vi "GeoData.vi"() -> ()   [LabVIEW 2017] (continued)
\n76008\t48367\tAledo\tTX\tParker County\tH1\n79035\t48369\tFriona\tTX\tParmer County\tH1\n79325\t48369\tFarwell\tTX\tParmer County\tH1\n79009\t48369\tBovina\tTX\tParmer County\tH1\n79347\t48369\tMuleshoe\tTX\tParmer County\tH1\n79053\t48369\tLazbuddie\tTX\tParmer County\tH1\n79740\t48371\tGirvin\tTX\tPecos County\tH1\n79735\t48371\tFort stockton\tTX\tPecos County\tH1\n79743\t48371\tImperial\tTX\tPecos County\tH1\n79781\t48371\tSheffield\tTX\tPecos County\tH1\n79730\t48371\tCoyanosa\tTX\tPecos County\tH1\n79744\t48371\tIraan\tTX\tPecos County\tH1\n77350\t48373\tLeggett\tTX\tPolk County\tH1\n77326\t48373\tAce\tTX\tPolk County\tH1\n75936\t48373\tChester\tTX\tPolk County\tH1\n77332\t48373\tDallardsville\tTX\tPolk County\tH1\n77327\t48373\tCleveland\tTX\tPolk County\tH1\n75960\t48373\tMoscow\tTX\tPolk County\tH1\n77360\t48373\tOnalaska\tTX\tPolk County\tH1\n77351\t48373\tLivingston\tTX\tPolk County\tH1\n75934\t48373\tCamden\tTX\tPolk County\tH1\n75939\t48373\tCorrigan\tTX\tPolk County\tH1\n77335\t48373\tGoodrich\tTX\tPolk County\tH1\n77399\t48373\tLivingston\tTX\tPolk County\tH1\n79103\t48375\tAmarillo\tTX\tPotter County\tH1\n79116\t48375\tAmarillo\tTX\tPotter County\tH1\n79012\t48375\tBushland\tTX\tPotter County\tH1\n79106\t48375\tAmarillo\tTX\tPotter County\tH1\n79102\t48375\tAmarillo\tTX\tPotter County\tH1\n79068\t48375\tPanhandle\tTX\tPotter County\tH1\n79108\t48375\tAmarillo\tTX\tPotter County\tH1\n79105\t48375\tAmarillo\tTX\tPotter County\tH1\n79107\t48375\tAmarillo\tTX\tPotter County\tH1\n79124\t48375\tAmarillo\tTX\tPotter County\tH1\n79159\t48375\tAmarillo\tTX\tPotter County\tH1\n79098\t48375\tWildorado\tTX\tPotter County\tH1\n79058\t48375\tMasterson\tTX\tPotter County\tH1\n79120\t48375\tAmarillo\tTX\tPotter County\tH1\n79117\t48375\tAmarillo\tTX\tPotter County\tH1\n79118\t48375\tAmarillo\tTX\tPotter County\tH1\n79111\t48375\tAmarillo\tTX\tPotter County\tH1\n79101\t48375\tAmarillo\tTX\tPotter County\tH1\n79109\t48375\tAmarillo\tTX\tPotter County\tH1\n79121\t48375\tAmarillo\tTX\tPotter County\tH1\n79104\t48375\tAmarillo\tTX\tPotter County\tH1\n79845\t48377\tPresidio\tTX\tPresidio County\tH1\n79843\t48377\tMarfa\tTX\tPresidio County\tH1\n79846\t48377\tRedford\tTX\tPresidio County\tH1\n75472\t48379\tPoint\tTX\tRains County\tH1\n75410\t48379\tAlba\tTX\tRains County\tH1\n75440\t48379\tEmory\tTX\tRains County\tH1\n75497\t48379\tYantis\tTX\tRains County\tH1\n75453\t48379\tLone oak\tTX\tRains County\tH1\n79103\t48381\tAmarillo\tTX\tRandall County\tH1\n79106\t48381\tAmarillo\tTX\tRandall County\tH1\n79124\t48381\tAmarillo\tTX\tRandall County\tH1\n79098\t48381\tWildorado\tTX\tRandall County\tH1\n79119\t48381\tAmarillo\tTX\tRandall County\tH1\n79016\t48381\tCanyon\tTX\tRandall County\tH1\n79042\t48381\tHappy\tTX\tRandall County\tH1\n79110\t48381\tAmarillo\tTX\tRandall County\tH1\n79118\t48381\tAmarillo\tTX\tRandall County\tH1\n79015\t48381\tCanyon\tTX\tRandall County\tH1\n79114\t48381\tAmarillo\tTX\tRandall County\tH1\n79091\t48381\tUmbarger\tTX\tRandall County\tH1\n79019\t48381\tClaude\tTX\tRandall County\tH1\n79109\t48381\tAmarillo\tTX\tRandall County\tH1\n79121\t48381\tAmarillo\tTX\tRandall County\tH1\n79094\t48381\tWayside\tTX\tRandall County\tH1\n79739\t48383\tGarden city\tTX\tReagan County\tH1\n76932\t48383\tBig lake\tTX\tReagan County\tH1\n78833\t48385\tCamp wood\tTX\tReal County\tH1\n78873\t48385\tLeakey\tTX\tReal County\tH1\n78828\t48385\tBarksdale\tTX\tReal County\tH1\n78879\t48385\tRio frio\tTX\tReal County\tH1\n75416\t48387\tBlossom\tTX\tRed River County\tH1\n75550\t48387\tAnnona\tTX\tRed River County\tH1\n75554\t48387\tAvery\tTX\tRed River County\tH1\n75435\t48387\tDeport\tTX\tRed River County\tH1\n75436\t48387\tDetroit\tTX\tRed River County\tH1\n75417\t48387\tBogata\tTX\tRed River County\tH1\n75412\t48387\tBagwell\tTX\tRed River County\tH1\n75426\t48387\tClarksville\tTX\tRed River County\tH1\n75559\t48387\tDe kalb\tTX\tRed River County\tH1\n79718\t48389\tBalmorhea\tTX\tReeves County\tH1\n79780\t48389\tSaragosa\tTX\tReeves County\tH1\n79785\t48389\tToyah\tTX\tReeves County\tH1\n79770\t48389\tOrla\tTX\tReeves County\tH1\n79772\t48389\tPecos\tTX\tReeves County\tH1\n77990\t48391\tTivoli\tTX\tRefugio County\tH1\n77950\t48391\tAustwell\tTX\tRefugio County\tH1\n78393\t48391\tWoodsboro\tTX\tRefugio County\tH1\n78340\t48391\tBayside\tTX\tRefugio County\tH1\n78377\t48391\tRefugio\tTX\tRefugio County\tH1\n79065\t48393\tPampa\tTX\tRoberts County\tH1\n79070\t48393\tPerryton\tTX\tRoberts County\tH1\n79059\t48393\tMiami\tTX\tRoberts County\tH1\n76629\t48395\tBremond\tTX\tRobertson County\tH1\n77856\t48395\tFranklin\tTX\tRobertson County\tH1\n77865\t48395\tMarquez\tTX\tRobertson County\tH1\n77867\t48395\tMumford\tTX\tRobertson County\tH1\n77870\t48395\tNew baden\tTX\tRobertson County\tH1\n77859\t48395\tHearne\tTX\tRobertson County\tH1\n77882\t48395\tWheelock\tTX\tRobertson County\tH1\n77807\t48395\tBryan\tTX\tRobertson County\tH1\n76653\t48395\tKosse\tTX\tRobertson County\tH1\n77837\t48395\tCalvert\tTX\tRobertson County\tH1\n77808\t48395\tBryan\tTX\tRobertson County\tH1\n76687\t48395\tThornton\tTX\tRobertson County\tH1\n75098\t48397\tWylie\tTX\tRockwall County\tH1\n75032\t48397\tRockwall\tTX\tRockwall County\tH1\n75088\t48397\tRowlett\tTX\tRockwall County\tH1\n75087\t48397\tRockwall\tTX\tRockwall County\tH1\n75089\t48397\tRowlett\tTX\tRockwall County\tH1\n75160\t48397\tTerrell\tTX\tRockwall County\tH1\n75126\t48397\tForney\tTX\tRockwall County\tH1\n75189\t48397\tRoyse city\tTX\tRockwall County\tH1\n75132\t48397\tFate\tTX\tRockwall County\tH1\n76821\t48399\tBallinger\tTX\tRunnels County\tH1\n79566\t48399\tWingate\tTX\tRunnels County\tH1\n76865\t48399\tNorton\tTX\tRunnels County\tH1\n79567\t48399\tWinters\tTX\tRunnels County\tH1\n76861\t48399\tMiles\tTX\tRunnels County\tH1\n76875\t48399\tRowena\tTX\tRunnels County\tH1\n79538\t48399\tNovice\tTX\tRunnels County\tH1\n76882\t48399\tTalpa\tTX\tRunnels County\tH1\n76933\t48399\tBronte\tTX\tRunnels County\tH1\n75669\t48401\tLong branch\tTX\tRusk County\tH1\n75680\t48401\tMinden\tTX\tRusk County\tH1\n75652\t48401\tHenderson\tTX\tRusk County\tH1\n75784\t48401\tReklaw\tTX\tRusk County\tH1\n75975\t48401\tTimpson\tTX\tRusk County\tH1\n75760\t48401\tCushing\tTX\tRusk County\tH1\n75681\t48401\tMount enterprise\tTX\tRusk County\tH1\n75689\t48401\tSelman city\tTX\tRusk County\tH1\n75667\t48401\tLaneville\tTX\tRusk County\tH1\n75650\t48401\tHallsville\tTX\tRusk County\tH1\n75666\t48401\tLaird hill\tTX\tRusk County\tH1\n75687\t48401\tPrice\tTX\tRusk County\tH1\n75691\t48401\tTatum\tTX\tRusk County\tH1\n75633\t48401\tCarthage\tTX\tRusk County\tH1\n75603\t48401\tLongview\tTX\tRusk County\tH1\n75631\t48401\tBeckville\tTX\tRusk County\tH1\n75654\t48401\tHenderson\tTX\tRusk County\tH1\n75946\t48401\tGarrison\tTX\tRusk County\tH1\n75662\t48401\tKilgore\tTX\tRusk County\tH1\n75684\t48401\tOverton\tTX\tRusk County\tH1\n75682\t48401\tNew london\tTX\tRusk County\tH1\n75658\t48401\tJoinerville\tTX\tRusk County\tH1\n75930\t48403\tBronson\tTX\tSabine County\tH1\n75948\t48403\tHemphill\tTX\tSabine County\tH1\n75968\t48403\tPineland\tTX\tSabine County\tH1\n75931\t48403\tBrookeland\tTX\tSabine County\tH1\n75972\t48403\tSan augustine\tTX\tSabine County\tH1\n75959\t48403\tMilam\tTX\tSabine County\tH1\n75929\t48405\tBroaddus\tTX\tSan Augustine County\tH1\n75930\t48405\tBronson\tTX\tSan Augustine County\tH1\n75935\t48405\tCenter\tTX\tSan Augustine County\tH1\n75972\t48405\tSan augustine\tTX\tSan Augustine County\tH1\n75961\t48405\tNacogdoches\tTX\tSan Augustine County\tH1\n77371\t48407\tShepherd\tTX\tSan Jacinto County\tH1\n77331\t48407\tColdspring\tTX\tSan Jacinto County\tH1\n77358\t48407\tNew waverly\tTX\tSan Jacinto County\tH1\n77320\t48407\tHuntsville\tTX\tSan Jacinto County\tH1\n77359\t48407\tOakhurst\tTX\tSan Jacinto County\tH1\n77327\t48407\tCleveland\tTX\tSan Jacinto County\tH1\n77328\t48407\tCleveland\tTX\tSan Jacinto County\tH1\n77378\t48407\tWillis\tTX\tSan Jacinto County\tH1\n77364\t48407\tPointblank\tTX\tSan Jacinto County\tH1\n78335\t48409\tAransas pass\tTX\tSan Patricio County\tH1\n78389\t48409\tSkidmore\tTX\tSan Patricio County\tH1\n78359\t48409\tGregory\tTX\tSan Patricio County\tH1\n78370\t48409\tOdem\tTX\tSan Patricio County\tH1\n78352\t48409\tEdroy\tTX\tSan Patricio County\tH1\n78368\t48409\tMathis\tTX\tSan Patricio County\tH1\n78362\t48409\tIngleside\tTX\tSan Patricio County\tH1\n78390\t48409\tTaft\tTX\tSan Patricio County\tH1\n78374\t48409\tPortland\tTX\tSan Patricio County\tH1\n78336\t48409\tAransas pass\tTX\tSan Patricio County\tH1\n78387\t48409\tSinton\tTX\tSan Patricio County\tH1\n76871\t48411\tRichland springs\tTX\tSan Saba County\tH1\n76872\t48411\tRochelle\tTX\tSan Saba County\tH1\n76832\t48411\tCherokee\tTX\tSan Saba County\tH1\n76877\t48411\tSan saba\tTX\tSan Saba County\tH1\n76936\t48413\tEldorado\tTX\tSchleicher County\tH1\n79512\t48415\tColorado city\tTX\tScurry County\tH1\n79532\t48415\tLoraine\tTX\tScurry County\tH1\n79526\t48415\tHermleigh\tTX\tScurry County\tH1\n79516\t48415\tDunn\tTX\tScurry County\tH1\n79549\t48415\tSnyder\tTX\tScurry County\tH1\n79517\t48415\tFluvanna\tTX\tScurry County\tH1\n79527\t48415\tIra\tTX\tScurry County\tH1\n79504\t48417\tBaird\tTX\tShackelford County\tH1\n79601\t48417\tAbilene\tTX\tShackelford County\tH1\n76430\t48417\tAlbany\tTX\tShackelford County\tH1\n76464\t48417\tMoran\tTX\tShackelford County\tH1\n79533\t48417\tLueders\tTX\tShackelford County\tH1\n75973\t48419\tShelbyville\tTX\tShelby County\tH1\n75975\t48419\tTimpson\tTX\tShelby County\tH1\n75935\t48419\tCenter\tTX\tShelby County\tH1\n75974\t48419\tTenaha\tTX\tShelby County\tH1\n75643\t48419\tGary\tTX\tShelby County\tH1\n75954\t48419\tJoaquin\tTX\tShelby County\tH1\n79022\t48421\tDalhart\tTX\tSherman County\tH1\n79084\t48421\tStratford\tTX\tSherman County\tH1\n73960\t48421\tTexhoma\tTX\tSherman County\tH1\n75704\t48423\tTyler\tTX\tSmith County\tH1\n75713\t48423\tTyler\tTX\tSmith County\tH1\n75762\t48423\tFlint\tTX\tSmith County\tH1\n75791\t48423\tWhitehouse\tTX\tSmith County\tH1\n75707\t48423\tTyler\tTX\tSmith County\tH1\n75712\t48423\tTyler\tTX\tSmith County\tH1\n75140\t48423\tGrand saline\tTX\tSmith County\tH1\n75773\t48423\tMineola\tTX\tSmith County\tH1\n75790\t48423\tVan\tTX\tSmith County\tH1\n75711\t48423\tTyler\tTX\tSmith County\tH1\n75708\t48423\tTyler\tTX\tSmith County\tH1\n75771\t48423\tLindale\tTX\tSmith County\tH1\n75710\t48423\tTyler\tTX\tSmith County\tH1\n75792\t48423\tWinona\tTX\tSmith County\tH1\n75709\t48423\tTyler\tTX\tSmith County\tH1\n75789\t48423\tTroup\tTX\tSmith County\tH1\n75750\t48423\tArp\tTX\tSmith County\tH1\n75705\t48423\tTyler\tTX\tSmith County\tH1\n75799\t48423\tTyler\tTX\tSmith County\tH1\n75798\t48423\tTyler\tTX\tSmith County\tH1\n75703\t48423\tTyler\tTX\tSmith County\tH1\n75706\t48423\tTyler\tTX\tSmith County\tH1\n75647\t48423\tGladewater\tTX\tSmith County\tH1\n75702\t48423\tTyler\tTX\tSmith County\tH1\n75662\t48423\tKilgore\tTX\tSmith County\tH1\n75684\t48423\tOverton\tTX\tSmith County\tH1\n75701\t48423\tTyler\tTX\tSmith County\tH1\n75757\t48423\tBullard\tTX\tSmith County\tH1\n76043\t48425\tGlen rose\tTX\tSomervell County\tH1\n76048\t48425\tGranbury\tTX\tSomervell County\tH1\n76033\t48425\tCleburne\tTX\tSomervell County\tH1\n76433\t48425\tBluff dale\tTX\tSomervell County\tH1\n76031\t48425\tCleburne\tTX\tSomervell County\tH1\n76077\t48425\tRainbow\tTX\tSomervell County\tH1\n76070\t48425\tNemo\tTX\tSomervell County\tH1\n78582\t48427\tRio grande city\tTX\tStarr County\tH1\n78584\t48427\tRoma\tTX\tStarr County\tH1\n78563\t48427\tLinn\tTX\tStarr County\tH1\n78536\t48427\tDelmita\tTX\tStarr County\tH1\n78585\t48427\tSalineno\tTX\tStarr County\tH1\n78591\t48427\tSanta elena\tTX\tStarr County\tH1\n78548\t48427\tGrulla\tTX\tStarr County\tH1\n78545\t48427\tFalcon heights\tTX\tStarr County\tH1\n78588\t48427\tSan isidro\tTX\tStarr County\tH1\n78547\t48427\tGarciasville\tTX\tStarr County\tH1\n78595\t48427\tSullivan city\tTX\tStarr County\tH1\n78361\t48427\tHebbronville\tTX\tStarr County\tH1\n76424\t48429\tBreckenridge\tTX\tStephens County\tH1\n76429\t48429\tCaddo\tTX\tStephens County\tH1\n76470\t48429\tRanger\tTX\tStephens County\tH1\n76437\t48429\tCisco\tTX\tStephens County\tH1\n76430\t48429\tAlbany\tTX\tStephens County\tH1\n76464\t48429\tMoran\tTX\tStephens County\tH1\n76450\t48429\tGraham\tTX\tStephens County\tH1\n76951\t48431\tSterling city\tTX\tSterling County\tH1\n79502\t48433\tAspermont\tTX\tStonewall County\tH1\n79540\t48433\tOld glory\tTX\tStonewall County\tH1\n76874\t48435\tRoosevelt\tTX\tSutton County\tH1\n76950\t48435\tSonora\tTX\tSutton County\tH1\n79042\t48437\tHappy\tTX\tSwisher County\tH1\n79088\t48437\tTulia\tTX\tSwisher County\tH1\n79052\t48437\tKress\tTX\tSwisher County\tH1\n79094\t48437\tWayside\tTX\tSwisher County\tH1\n76114\t48439\tFort worth\tTX\tTarrant County\tH1\n76118\t48439\tFort worth\tTX\tTarrant County\tH1\n76179\t48439\tFort worth\tTX\tTarrant County\tH1\n76011\t48439\tArlington\tTX\tTarrant County\tH1\n76015\t48439\tArlington\tTX\tTarrant County\tH1\n76007\t48439\tArlington\tTX\tTarrant County\tH1\n76096\t48439\tArlington\tTX\tTarrant County\tH1\n76161\t48439\tFort worth\tTX\tTarrant County\tH1\n76039\t48439\tEuless\tTX\tTarrant County\tH1\n76051\t48439\tGrapevine\tTX\tTarrant County\tH1\n76054\t48439\tHurst\tTX\tTarrant County\tH1\n76108\t48439\tFort worth\tTX\tTarrant County\tH1\n76115\t48439\tFort worth\tTX\tTarrant County\tH1\n76103\t48439\tFort worth\tTX\tTarrant County\tH1\n76107\t48439\tFort worth\tTX\tTarrant County\tH1\n76135\t48439\tFort worth\tTX\tTarrant County\tH1\n76133\t48439\tFort worth\tTX\tTarrant County\tH1\n76155\t48439\tFort worth\tTX\tTarrant County\tH1\n76262\t48439\tRoanoke\tTX\tTarrant County\tH1\n76180\t48439\tNorth richland hills\tTX\tTarrant County\tH1\n76010\t48439\tArlington\tTX\tTarrant County\tH1\n76014\t48439\tArlington\tTX\tTarrant County\tH1\n76016\t48439\tArlington\tTX\tTarrant County\tH1\n76163\t48439\tFort worth\tTX\tTarrant County\tH1\n76162\t48439\tFort worth\tTX\tTarrant County\tH1\n76122\t48439\tFort worth\tTX\tTarrant County\tH1\n76040\t48439\tEuless\tTX\tTarrant County\tH1\n76109\t48439\tFort worth\tTX\tTarrant County\tH1\n76123\t48439\tFort worth\tTX\tTarrant County\tH1\n76131\t48439\tFort worth\tTX\tTarrant County\tH1\n76137\t48439\tFort worth\tTX\tTarrant County\tH1\n76106\t48439\tFort worth\tTX\tTarrant County\tH1\n76099\t48439\tGrapevine\tTX\tTarrant County\tH1\n76148\t48439\tFort worth\tTX\tTarrant County\tH1\n76182\t48439\tNorth richland hills\tTX\tTarrant County\tH1\n76177\t48439\tFort worth\tTX\tTarrant County\tH1\n76002\t48439\tArlington\tTX\tTarrant County\tH1\n76020\t48439\tAzle\tTX\tTarrant County\tH1\n76185\t48439\tFort worth\tTX\tTarrant County\tH1\n76127\t48439\tNaval air station jrb\tTX\tTarrant County\tH1\n76190\t48439\tFort worth\tTX\tTarrant County\tH1\n76191\t48439\tFort worth\tTX\tTarrant County\tH1\n76199\t48439\tFort worth\tTX\tTarrant County\tH1\n76195\t48439\tFort worth\tTX\tTarrant County\tH1\n75050\t48439\tGrand prairie\tTX\tTarrant County\tH1\n75051\t48439\tGrand prairie\tTX\tTarrant County\tH1\n76092\t48439\tSouthlake\tTX\tTarrant County\tH1\n76119\t48439\tFort worth\tTX\tTarrant County\tH1\n76101\t48439\tFort worth\tTX\tTarrant County\tH1\n76164\t48439\tFort worth\tTX\tTarrant County\tH1\n76001\t48439\tArlington\tTX\tTarrant County\tH1\n76017\t48439\tArlington\tTX\tTarrant County\tH1\n76021\t48439\tBedford\tTX\tTarrant County\tH1\n76004\t48439\tArlington\tTX\tTarrant County\tH1\n75261\t48439\tDallas\tTX\tTarrant County\tH1\n76003\t48439\tArlington\tTX\tTarrant County\tH1\n76193\t48439\tFort worth\tTX\tTarrant County\tH1\n75053\t48439\tGrand prairie\tTX\tTarrant County\tH1\n76034\t48439\tColleyville\tTX\tTarrant County\tH1\n76036\t48439\tCrowley\tTX\tTarrant County\tH1\n76104\t48439\tFort worth\tTX\tTarrant County\tH1\n76120\t48439\tFort worth\tTX\tTarrant County\tH1\n76006\t48439\tArlington\tTX\tTarrant County\tH1\n76018\t48439\tArlington\tTX\tTarrant County\tH1\n76022\t48439\tBedford\tTX\tTarrant County\tH1\n76095\t48439\tBedford\tTX\tTarrant County\tH1\n76130\t48439\tFort worth\tTX\tTarrant County\tH1\n75028\t48439\tFlower mound\tTX\tTarrant County\tH1\n76105\t48439\tFort worth\tTX\tTarrant County\tH1\n76111\t48439\tFort worth\tTX\tTarrant County\tH1\n76140\t48439\tFort worth\tTX\tTarrant County\tH1\n76110\t48439\tFort worth\tTX\tTarrant County\tH1\n76124\t48439\tFort worth\tTX\tTarrant County\tH1\n76147\t48439\tFort worth\tTX\tTarrant County\tH1\n76136\t48439\tFort worth\tTX\tTarrant County\tH1\n76192\t48439\tFort worth\tTX\tTarrant County\tH1\n76129\t48439\tFort worth\tTX\tTarrant County\tH1\n76019\t48439\tArlington\tTX\tTarrant County\tH1\n75022\t48439\tFlower mound\tTX\tTarrant County\tH1\n75054\t48439\tGrand prairie\tTX\tTarrant County\tH1\n76052\t48439\tHaslet\tTX\tTarrant County\tH1\n76063\t48439\tMansfield\tTX\tTarrant County\tH1\n76053\t48439\tHurst\tTX\tTarrant County\tH1\n76116\t48439\tFort worth\tTX\tTarrant County\tH1\n76121\t48439\tFort worth\tTX\tTarrant County\tH1\n76134\t48439\tFort worth\tTX\tTarrant County\tH1\n76132\t48439\tFort worth\tTX\tTarrant County\tH1\n76244\t48439\tKeller\tTX\tTarrant County\tH1\n76012\t48439\tArlington\tTX\tTarrant County\tH1\n76013\t48439\tArlington\tTX\tTarrant County\tH1\n76005\t48439\tArlington\tTX\tTarrant County\tH1\n76071\t48439\tNewark\tTX\tTarrant County\tH1\n76196\t48439\tFort worth\tTX\tTarrant County\tH1\n75052\t48439\tGrand prairie\tTX\tTarrant County\tH1\n76028\t48439\tBurleson\tTX\tTarrant County\tH1\n76060\t48439\tKennedale\tTX\tTarrant County\tH1\n76112\t48439\tFort worth\tTX\tTarrant County\tH1\n76117\t48439\tHaltom city\tTX\tTarrant County\tH1\n76102\t48439\tFort worth\tTX\tTarrant County\tH1\n76126\t48439\tFort worth\tTX\tTarrant County\tH1\n76248\t48439\tKeller\tTX\tTarrant County\tH1\n76008\t48439\tAledo\tTX\tTarrant County\tH1\n76094\t48439\tArlington\tTX\tTarrant County\tH1\n76113\t48439\tFort worth\tTX\tTarrant County\tH1\n76197\t48439\tFort worth\tTX\tTarrant County\tH1\n79536\t48441\tMerkel\tTX\tTaylor County\tH1\n79541\t48441\tOvalo\tTX\tTaylor County\tH1\n79697\t48441\tAbilene\tTX\tTaylor County\tH1\n79566\t48441\tWingate\tTX\tTaylor County\tH1\n79698\t48441\tAbilene\tTX\tTaylor County\tH1\n79601\t48441\tAbilene\tTX\tTaylor County\tH1\n79562\t48441\tTuscola\tTX\tTaylor County\tH1\n79561\t48441\tTrent\tTX\tTaylor County\tH1\n79608\t48441\tAbilene\tTX\tTaylor County\tH1\n79567\t48441\tWinters\tTX\tTaylor County\tH1\n79605\t48441\tAbilene\tTX\tTaylor County\tH1\n79607\t48441\tDyess afb\tTX\tTaylor County\tH1\n79530\t48441\tLawn\tTX\tTaylor County\tH1\n79508\t48441\tBuffalo gap\tTX\tTaylor County\tH1\n79519\t48441\tGoldsboro\tTX\tTaylor County\tH1\n79603\t48441\tAbilene\tTX\tTaylor County\tH1\n79606\t48441\tAbilene\tTX\tTaylor County\tH1\n79602\t48441\tAbilene\tTX\tTaylor County\tH1\n79604\t48441\tAbilene\tTX\tTaylor County\tH1\n79563\t48441\tTye\tTX\tTaylor County\tH1\n79699\t48441\tAbilene\tTX\tTaylor County\tH1\n79735\t48443\tFort stockton\tTX\tTerrell County\tH1\n79848\t48443\tSanderson\tTX\tTerrell County\tH1\n78851\t48443\tDryden\tTX\tTerrell County\tH1\n79359\t48445\tSeagraves\tTX\tTerry County\tH1\n79376\t48445\tTokio\tTX\tTerry County\tH1\n79373\t48445\tTahoka\tTX\tTerry County\tH1\n79378\t48445\tWellman\tTX\tTerry County\tH1\n79345\t48445\tMeadow\tTX\tTerry County\tH1\n79355\t48445\tPlains\tTX\tTerry County\tH1\n79316\t48445\tBrownfield\tTX\tTerry County\tH1\n76372\t48447\tNewcastle\tTX\tThrockmorton County\tH1\n76374\t48447\tOlney\tTX\tThrockmorton County\tH1\n76491\t48447\tWoodson\tTX\tThrockmorton County\tH1\n76430\t48447\tAlbany\tTX\tThrockmorton County\tH1\n76483\t48447\tThrockmorton\tTX\tThrockmorton County\tH1\n75493\t48449\tWinfield\tTX\tTitus County\tH1\n75455\t48449\tMount pleasant\tTX\tTitus County\tH1\n75558\t48449\tCookville\tTX\tTitus County\tH1\n75571\t48449\tOmaha\tTX\tTitus County\tH1\n75686\t48449\tPittsburg\tTX\tTitus County\tH1\n75487\t48449\tTalco\tTX\tTitus County\tH1\n75456\t48449\tMount pleasant\tTX\tTitus County\tH1\n76939\t48451\tKnickerbocker\tTX\tTom Green County\tH1\n76886\t48451\tVeribest\tTX\tTom Green County\tH1\n76935\t48451\tChristoval\tTX\tTom Green County\tH1\n76909\t48451\tSan angelo\tTX\tTom Green County\tH1\n76902\t48451\tSan angelo\tTX\tTom Green County\tH1\n76904\t48451\tSan angelo\tTX\tTom Green County\tH1\n76905\t48451\tSan angelo\tTX\tTom Green County\tH1\n76934\t48451\tCarlsbad\tTX\tTom Green County\tH1\n76861\t48451\tMiles\tTX\tTom Green County\tH1\n76940\t48451\tMereta\tTX\tTom Green County\tH1\n76937\t48451\tEola\tTX\tTom Green County\tH1\n76957\t48451\tWall\tTX\tTom Green County\tH1\n76906\t48451\tSan angelo\tTX\tTom Green County\tH1\n76901\t48451\tSan angelo\tTX\tTom Green County\tH1\n76903\t48451\tSan angelo\tTX\tTom Green County\tH1\n76955\t48451\tVancourt\tTX\tTom Green County\tH1\n76908\t48451\tGoodfellow afb\tTX\tTom Green County\tH1\n76958\t48451\tWater valley\tTX\tTom Green County\tH1\n78641\t48453\tLeander\tTX\tTravis County\tH1\n78758\t48453\tAustin\tTX\tTravis County\tH1\n78759\t48453\tAustin\tTX\tTravis County\tH1\n78751\t48453\tAustin\tTX\tTravis County\tH1\n78747\t48453\tAustin\tTX\tTravis County\tH1\n78722\t48453\tAustin\tTX\tTravis County\tH1\n78702\t48453\tAustin\tTX\tTravis County\tH1\n78725\t48453\tAustin\tTX\tTravis County\tH1\n78729\t48453\tAustin\tTX\tTravis County\tH1\n78741\t48453\tAustin\tTX\tTravis County\tH1\n78734\t48453\tAustin\tTX\tTravis County\tH1\n78716\t48453\tAustin\tTX\tTravis County\tH1\n78768\t48453\tAustin\tTX\tTravis County\tH1\n73301\t48453\tAustin\tTX\tTravis County\tH1\n76574\t48453\tTaylor\tTX\tTravis County\tH1\n78616\t48453\tDale\tTX\tTravis County\tH1\n78763\t48453\tAustin\tTX\tTravis County\tH1\n78757\t48453\tAustin\tTX\tTravis County\tH1\n78719\t48453\tAustin\tTX\tTravis County\tH1\n78738\t48453\tAustin\tTX\tTravis County\tH1\n78765\t48453\tAustin\tTX\tTravis County\tH1\n78778\t48453\tAustin\tTX\tTravis County\tH1\n78612\t48453\tCedar creek\tTX\tTravis County\tH1\n78652\t48453\tManchaca\tTX\tTravis County\tH1\n78753\t48453\tAustin\tTX\tTravis County\tH1\n78766\t48453\tAustin\tTX\tTravis County\tH1\n78767\t48453\tAustin\tTX\tTravis County\tH1\n78705\t48453\tAustin\tTX\tTravis County\tH1\n78724\t48453\tAustin\tTX\tTravis County\tH1\n78704\t48453\tAustin\tTX\tTravis County\tH1\n78709\t48453\tAustin\tTX\tTravis County\tH1\n78728\t48453\tAustin\tTX\tTravis County\tH1\n78714\t48453\tAustin\tTX\tTravis County\tH1\n78755\t48453\tAustin\tTX\tTravis County\tH1\n78742\t48453\tAustin\tTX\tTravis County\tH1\n78799\t48453\tAustin\tTX\tTravis County\tH1\n78779\t48453\tAustin\tTX\tTravis County\tH1\n78774\t48453\tAustin\tTX\tTravis County\tH1\n78634\t48453\tHutto\tTX\tTravis County\tH1\n78642\t48453\tLiberty hill\tTX\tTravis County\tH1\n78620\t48453\tDripping springs\tTX\tTravis County\tH1\n78617\t48453\tDel valle\tTX\tTravis County\tH1\n78750\t48453\tAustin\tTX\tTravis County\tH1\n78761\t48453\tAustin\tTX\tTravis County\tH1\n78744\t48453\tAustin\tTX\tTravis County\tH1\n78723\t48453\tAustin\tTX\tTravis County\tH1\n78701\t48453\tAustin\tTX\tTravis County\tH1\n78736\t48453\tAustin\tTX\tTravis County\tH1\n78732\t48453\tAustin\tTX\tTravis County\tH1\n78764\t48453\tAustin\tTX\tTravis County\tH1\n78772\t48453\tAustin\tTX\tTravis County\tH1\n78654\t48453\tMarble falls\tTX\tTravis County\tH1\n78615\t48453\tCoupland\tTX\tTravis County\tH1\n78640\t48453\tKyle\tTX\tTravis County\tH1\n78610\t48453\tBuda\tTX\tTravis County\tH1\n78663\t48453\tRound mountain\tTX\tTravis County\tH1\n78645\t48453\tLeander\tTX\tTravis County\tH1\n78749\t48453\tAustin\tTX\tTravis County\tH1\n78752\t48453\tAustin\tTX\tTravis County\tH1\n78708\t48453\tAustin\tTX\tTravis County\tH1\n78712\t48453\tAustin\tTX\tTravis County\tH1\n78713\t48453\tAustin\tTX\tTravis County\tH1\n78730\t48453\tAustin\tTX\tTravis County\tH1\n78711\t48453\tAustin\tTX\tTravis County\tH1\n78762\t48453\tAustin\tTX\tTravis County\tH1\n78613\t48453\tCedar park\tTX\tTravis County\tH1\n78664\t48453\tRound rock\tTX\tTravis County\tH1\n78756\t48453\tAustin\tTX\tTravis County\tH1\n78745\t48453\tAustin\tTX\tTravis County\tH1\n78727\t48453\tAustin\tTX\tTravis County\tH1\n78720\t48453\tAustin\tTX\tTravis County\tH1\n78733\t48453\tAustin\tTX\tTravis County\tH1\n78739\t48453\tAustin\tTX\tTravis County\tH1\n78691\t48453\tPflugerville\tTX\tTravis County\tH1\n78718\t48453\tAustin\tTX\tTravis County\tH1\n78621\t48453\tElgin\tTX\tTravis County\tH1\n78748\t48453\tAustin\tTX\tTravis County\tH1\n78669\t48453\tSpicewood\tTX\tTravis County\tH1\n78721\t48453\tAustin\tTX\tTravis County\tH1\n78735\t48453\tAustin\tTX\tTravis County\tH1\n78737\t48453\tAustin\tTX\tTravis County\tH1\n78731\t48453\tAustin\tTX\tTravis County\tH1\n78760\t48453\tAustin\tTX\tTravis County\tH1\n78660\t48453\tPflugerville\tTX\tTravis County\tH1\n78653\t48453\tManor\tTX\tTravis County\tH1\n78746\t48453\tAustin\tTX\tTravis County\tH1\n78754\t48453\tAustin\tTX\tTravis County\tH1\n78703\t48453\tAustin\tTX\tTravis County\tH1\n78726\t48453\tAustin\tTX\tTravis County\tH1\n78715\t48453\tAustin\tTX\tTravis County\tH1\n78710\t48453\tAustin\tTX\tTravis County\tH1\n75862\t48455\tTrinity\tTX\tTrinity County\tH1\n75847\t48455\tKennard\tTX\tTrinity County\tH1\n75865\t48455\tWoodlake\tTX\tTrinity County\tH1\n75904\t48455\tLufkin\tTX\tTrinity County\tH1\n75856\t48455\tPennington\tTX\tTrinity County\tH1\n75834\t48455\tCentralia\tTX\tTrinity County\tH1\n75926\t48455\tApple springs\tTX\tTrinity County\tH1\n75845\t48455\tGroveton\tTX\tTrinity County\tH1\n75936\t48457\tChester\tTX\tTyler County\tH1\n75942\t48457\tDoucette\tTX\tTyler County\tH1\n75990\t48457\tWoodville\tTX\tTyler County\tH1\n75938\t48457\tColmesneil\tTX\tTyler County\tH1\n77624\t48457\tHillister\tTX\tTyler County\tH1\n77660\t48457\tSpurger\tTX\tTyler County\tH1\n77664\t48457\tWarren\tTX\tTyler County\tH1\n75979\t48457\tWoodville\tTX\tTyler County\tH1\n77616\t48457\tFred\tTX\tTyler County\tH1\n75605\t48459\tLongview\tTX\tUpshur County\tH1\n75604\t48459\tLongview\tTX\tUpshur County\tH1\n75765\t48459\tHawkins\tTX\tUpshur County\tH1\n75755\t48459\tBig sandy\tTX\tUpshur County\tH1\n75451\t48459\tLeesburg\tTX\tUpshur County\tH1\n75644\t48459\tGilmer\tTX\tUpshur County\tH1\n75494\t48459\tWinnsboro\tTX\tUpshur County\tH1\n75686\t48459\tPittsburg\tTX\tUpshur County\tH1\n75683\t48459\tOre city\tTX\tUpshur County\tH1\n75645\t48459\tGilmer\tTX\tUpshur County\tH1\n75640\t48459\tDiana\tTX\tUpshur County\tH1\n75647\t48459\tGladewater\tTX\tUpshur County\tH1\n75693\t48459\tWhite oak\tTX\tUpshur County\tH1\n79755\t48461\tMidkiff\tTX\tUpton County\tH1\n79778\t48461\tRankin\tTX\tUpton County\tH1\n79752\t48461\tMc camey\tTX\tUpton County\tH1\n78833\t48463\tCamp wood\tTX\tUvalde County\tH1\n78802\t48463\tUvalde\tTX\tUvalde County\tH1\n78870\t48463\tKnippa\tTX\tUvalde County\tH1\n78838\t48463\tConcan\tTX\tUvalde County\tH1\n78881\t48463\tSabinal\tTX\tUvalde County\tH1\n78884\t48463\tUtopia\tTX\tUvalde County\tH1\n78801\t48463\tUvalde\tTX\tUvalde County\tH1\n78842\t48465\tDel rio\tTX\tVal Verde County\tH1\n78847\t48465\tDel rio\tTX\tVal Verde County\tH1\n78840\t48465\tDel rio\tTX\tVal Verde County\tH1\n78837\t48465\tComstock\tTX\tVal Verde County\tH1\n78841\t48465\tDel rio\tTX\tVal Verde County\tH1\n78871\t48465\tLangtry\tTX\tVal Verde County\tH1\n78843\t48465\tLaughlin afb\tTX\tVal Verde County\tH1\n75474\t48467\tQuinlan\tTX\tVan Zandt County\tH1\n75103\t48467\tCanton\tTX\tVan Zandt County\tH1\n75117\t48467\tEdgewood\tTX\tVan Zandt County\tH1\n75140\t48467\tGrand saline\tTX\tVan Zandt County\tH1\n75169\t48467\tWills point\tTX\tVan Zandt County\tH1\n75773\t48467\tMineola\tTX\tVan Zandt County\tH1\n75778\t48467\tMurchison\tTX\tVan Zandt County\tH1\n75790\t48467\tVan\tTX\tVan Zandt County\tH1\n75127\t48467\tFruitvale\tTX\tVan Zandt County\tH1\n75124\t48467\tEustace\tTX\tVan Zandt County\tH1\n75754\t48467\tBen wheeler\tTX\tVan Zandt County\tH1\n75758\t48467\tChandler\tTX\tVan Zandt County\tH1\n75147\t48467\tMabank\tTX\tVan Zandt County\tH1\n75752\t48467\tAthens\tTX\tVan Zandt County\tH1\n75756\t48467\tBrownsboro\tTX\tVan Zandt County\tH1\n77979\t48469\tPort lavaca\tTX\tVictoria County\tH1\n77976\t48469\tNursery\tTX\tVictoria County\tH1\n77904\t48469\tVictoria\tTX\tVictoria County\tH1\n77951\t48469\tBloomington\tTX\tVictoria County\tH1\n77988\t48469\tTelferner\tTX\tVictoria County\tH1\n77974\t48469\tMeyersville\tTX\tVictoria County\tH1\n77901\t48469\tVictoria\tTX\tVictoria County\tH1\n77973\t48469\tMcfaddin\tTX\tVictoria County\tH1\n77995\t48469\tYoakum\tTX\tVictoria County\tH1\n77968\t48469\tInez\tTX\tVictoria County\tH1\n77902\t48469\tVictoria\tTX\tVictoria County\tH1\n77905\t48469\tVictoria\tTX\tVictoria County\tH1\n77977\t48469\tPlacedo\tTX\tVictoria County\tH1\n77903\t48469\tVictoria\tTX\tVictoria County\tH1\n75862\t48471\tTrinity\tTX\tWalker County\tH1\n77358\t48471\tNew waverly\tTX\tWalker County\tH1\n77340\t48471\tHuntsville\tTX\tWalker County\tH1\n77320\t48471\tHuntsville\tTX\tWalker County\tH1\n77341\t48471\tHuntsville\tTX\tWalker County\tH1\n77367\t48471\tRiverside\tTX\tWalker County\tH1\n75852\t48471\tMidway\tTX\tWalker County\tH1\n77342\t48471\tHuntsville\tTX\tWalker County\tH1\n77378\t48471\tWillis\tTX\tWalker County\tH1\n77318\t48471\tWillis\tTX\tWalker County\tH1\n77873\t48471\tRichards\tTX\tWalker County\tH1\n77831\t48471\tBedias\tTX\tWalker County\tH1\n77334\t48471\tDodge\tTX\tWalker County\tH1\n77466\t48473\tPattison\tTX\tWaller County\tH1\n77355\t48473\tMagnolia\tTX\tWaller County\tH1\n77493\t48473\tKaty\tTX\tWaller County\tH1\n77868\t48473\tNavasota\tTX\tWaller County\tH1\n77423\t48473\tBrookshire\tTX\tWaller County\tH1\n77445\t48473\tHempstead\tTX\tWaller County\tH1\n77447\t48473\tHockley\tTX\tWaller County\tH1\n77363\t48473\tPlantersville\tTX\tWaller County\tH1\n77484\t48473\tWaller\tTX\tWaller County\tH1\n77494\t48473\tKaty\tTX\tWaller County\tH1\n77446\t48473\tPrairie view\tTX\tWaller County\tH1\n79777\t48475\tPyote\tTX\tWard County\tH1\n79742\t48475\tGrandfalls\tTX\tWard County\tH1\n79719\t48475\tBarstow\tTX\tWard County\tH1\n79756\t48475\tMonahans\tTX\tWard County\tH1\n79788\t48475\tWickett\tTX\tWard County\tH1\n77833\t48477\tBrenham\tTX\tWashington County\tH1\n78932\t48477\tCarmine\tTX\tWashington County\tH1\n77868\t48477\tNavasota\tTX\tWashington County\tH1\n78946\t48477\tLedbetter\tTX\tWashington County\tH1\n77835\t48477\tBurton\tTX\tWashington County\tH1\n77880\t48477\tWashington\tTX\tWashington County\tH1\n77426\t48477\tChappell hill\tTX\tWashington County\tH1\n77834\t48477\tBrenham\tTX\tWashington County\tH1\n78045\t48479\tLaredo\tTX\tWebb County\tH1\n78344\t48479\tBruni\tTX\tWebb County\tH1\n78044\t48479\tLaredo\tTX\tWebb County\tH1\n78041\t48479\tLaredo\tTX\tWebb County\tH1\n78040\t48479\tLaredo\tTX\tWebb County\tH1\n78042\t48479\tLaredo\tTX\tWebb County\tH1\n78371\t48479\tOilton\tTX\tWebb County\tH1\n78046\t48479\tLaredo\tTX\tWebb County\tH1\n78043\t48479\tLaredo\tTX\tWebb County\tH1\n78369\t48479\tMirando city\tTX\tWebb County\tH1\n77488\t48481\tWharton\tTX\tWharton County\tH1\n77448\t48481\tHungerford\tTX\tWharton County\tH1\n77436\t48481\tEgypt\tTX\tWharton County\tH1\n77435\t48481\tEast bernard\tTX\tWharton County\tH1\n77420\t48481\tBoling\tTX\tWharton County\tH1\n77455\t48481\tLouise\tTX\tWharton County\tH1\n77434\t48481\tEagle lake\tTX\tWharton County\tH1\n77437\t48481\tEl campo\tTX\tWharton County\tH1\n77443\t48481\tGlen flora\tTX\tWharton County\tH1\n77467\t48481\tPierce\tTX\tWharton County\tH1\n77453\t48481\tLane city\tTX\tWharton County\tH1\n77454\t48481\tLissie\tTX\tWharton County\tH1\n77485\t48481\tWallis\tTX\tWharton County\tH1\n77432\t48481\tDanevang\tTX\tWharton County\tH1\n79079\t48483\tShamrock\tTX\tWheeler County\tH1\n79014\t48483\tCanadian\tTX\tWheeler County\tH1\n79057\t48483\tMclean\tTX\tWheeler County\tH1\n79011\t48483\tBriscoe\tTX\tWheeler County\tH1\n79003\t48483\tAllison\tTX\tWheeler County\tH1\n79061\t48483\tMobeetie\tTX\tWheeler County\tH1\n79096\t48483\tWheeler\tTX\tWheeler County\tH1\n76301\t48485\tWichita falls\tTX\tWichita County\tH1\n76305\t48485\tWichita falls\tTX\tWichita County\tH1\n76367\t48485\tIowa park\tTX\tWichita County\tH1\n76360\t48485\tElectra\tTX\tWichita County\tH1\n76307\t48485\tWichita falls\tTX\tWichita County\tH1\n76310\t48485\tWichita falls\tTX\tWichita County\tH1\n76302\t48485\tWichita falls\tTX\tWichita County\tH1\n76369\t48485\tKamay\tTX\tWichita County\tH1\n76309\t48485\tWichita falls\tTX\tWichita County\tH1\n76306\t48485\tWichita falls\tTX\tWichita County\tH1\n76354\t48485\tBurkburnett\tTX\tWichita County\tH1\n76308\t48485\tWichita falls\tTX\tWichita County\tH1\n76311\t48485\tSheppard afb\tTX\tWichita County\tH1\n76360\t48487\tElectra\tTX\tWilbarger County\tH1\n76364\t48487\tHarrold\tTX\tWilbarger County\tH1\n76384\t48487\tVernon\tTX\tWilbarger County\tH1\n79247\t48487\tOdell\tTX\tWilbarger County\tH1\n76373\t48487\tOklaunion\tTX\tWilbarger County\tH1\n79225\t48487\tChillicothe\tTX\tWilbarger County\tH1\n78569\t48489\tLyford\tTX\tWillacy County\tH1\n78590\t48489\tSan perlita\tTX\tWillacy County\tH1\n78550\t48489\tHarlingen\tTX\tWillacy County\tH1\n78561\t48489\tLasara\tTX\tWillacy County\tH1\n78594\t48489\tSebastian\tTX\tWillacy County\tH1\n78580\t48489\tRaymondville\tTX\tWillacy County\tH1\n78598\t48489\tPort mansfield\tTX\tWillacy County\tH1\n78633\t48491\tGeorgetown\tTX\tWilliamson County\tH1\n78641\t48491\tLeander\tTX\tWilliamson County\tH1\n78759\t48491\tAustin\tTX\tWilliamson County\tH1\n78729\t48491\tAustin\tTX\tWilliamson County\tH1\n78605\t48491\tBertram\tTX\tWilliamson County\tH1\n76574\t48491\tTaylor\tTX\tWilliamson County\tH1\n76577\t48491\tThorndale\tTX\tWilliamson County\tH1\n76578\t48491\tThrall\tTX\tWilliamson County\tH1\n76537\t48491\tJarrell\tTX\tWilliamson County\tH1\n78681\t48491\tRound rock\tTX\tWilliamson County\tH1\n78682\t48491\tRound rock\tTX\tWilliamson County\tH1\n76530\t48491\tGranger\tTX\tWilliamson County\tH1\n78717\t48491\tAustin\tTX\tWilliamson County\tH1\n78728\t48491\tAustin\tTX\tWilliamson County\tH1\n76571\t48491\tSalado\tTX\tWilliamson County\tH1\n76527\t48491\tFlorence\tTX\tWilliamson County\tH1\n76573\t48491\tSchwertner\tTX\tWilliamson County\tH1\n78634\t48491\tHutto\tTX\tWilliamson County\tH1\n78642\t48491\tLiberty hill\tTX\tWilliamson County\tH1\n78750\t48491\tAustin\tTX\tWilliamson County\tH1\n78646\t48491\tLeander\tTX\tWilliamson County\tH1\n78673\t48491\tWalburg\tTX\tWilliamson County\tH1\n78628\t48491\tGeorgetown\tTX\tWilliamson County\tH1\n78615\t48491\tCoupland\tTX\tWilliamson County\tH1\n78665\t48491\tRound rock\tTX\tWilliamson County\tH1\n78680\t48491\tRound rock\tTX\tWilliamson County\tH1\n78613\t48491\tCedar park\tTX\tWilliamson County\tH1\n78664\t48491\tRound rock\tTX\tWilliamson County\tH1\n78727\t48491\tAustin\tTX\tWilliamson County\tH1\n78627\t48491\tGeorgetown\tTX\tWilliamson County\tH1\n78674\t48491\tWeir\tTX\tWilliamson County\tH1\n78621\t48491\tElgin\tTX\tWilliamson County\tH1\n78630\t48491\tCedar park\tTX\tWilliamson County\tH1\n78683\t48491\tRound rock\tTX\tWilliamson County\tH1\n76511\t48491\tBartlett\tTX\tWilliamson County\tH1\n78626\t48491\tGeorgetown\tTX\tWilliamson County\tH1\n78660\t48491\tPflugerville\tTX\tWilliamson County\tH1\n78651\t48491\tMc neil\tTX\tWilliamson County\tH1\n78113\t48493\tFalls city\tTX\tWilson County\tH1\n78117\t48493\tHobson\tTX\tWilson County\tH1\n78161\t48493\tSutherland springs\tTX\tWilson County\tH1\n78114\t48493\tFloresville\tTX\tWilson County\tH1\n78064\t48493\tPleasanton\tTX\tWilson County\tH1\n78101\t48493\tAdkins\tTX\tWilson County\tH1\n78160\t48493\tStockdale\tTX\tWilson County\tH1\n78152\t48493\tSaint hedwig\tTX\tWilson County\tH1\n78112\t48493\tElmendorf\tTX\tWilson County\tH1\n78223\t48493\tSan antonio\tTX\tWilson County\tH1\n78147\t48493\tPoth\tTX\tWilson County\tH1\n78121\t48493\tLa vernia\tTX\tWilson County\tH1\n78140\t48493\tNixon\tTX\tWilson County\tH1\n78143\t48493\tPandora\tTX\tWilson County\tH1\n79789\t48495\tWink\tTX\tWinkler County\tH1\n79745\t48495\tKermit\tTX\tWinkler County\tH1\n76073\t48497\tParadise\tTX\tWise County\tH1\n76259\t48497\tPonder\tTX\tWise County\tH1\n76225\t48497\tAlvord\tTX\tWise County\tH1\n76246\t48497\tGreenwood\tTX\tWise County\tH1\n76078\t48497\tRhome\tTX\tWise County\tH1\n76020\t48497\tAzle\tTX\tWise County\tH1\n76487\t48497\tPoolville\tTX\tWise County\tH1\n76267\t48497\tSlidell\tTX\tWise County\tH1\n76023\t48497\tBoyd\tTX\tWise County\tH1\n76082\t48497\tSpringtown\tTX\tWise County\tH1\n76234\t48497\tDecatur\tTX\tWise County\tH1\n76247\t48497\tJustin\tTX\tWise County\tH1\n76426\t48497\tBridgeport\tTX\tWise County\tH1\n76249\t48497\tKrum\tTX\tWise County\tH1\n76270\t48497\tSunset\tTX\tWise County\tH1\n76431\t48497\tChico\tTX\tWise County\tH1\n76052\t48497\tHaslet\tTX\tWise County\tH1\n76239\t48497\tForestburg\tTX\tWise County\tH1\n76071\t48497\tNewark\tTX\tWise County\tH1\n76458\t48497\tJacksboro\tTX\tWise County\tH1\n75431\t48499\tComo\tTX\tWood County\tH1\n75410\t48499\tAlba\tTX\tWood County\tH1\n75765\t48499\tHawkins\tTX\tWood County\tH1\n75440\t48499\tEmory\tTX\tWood County\tH1\n75480\t48499\tScroggins\tTX\tWood County\tH1\n75497\t48499\tYantis\tTX\tWood County\tH1\n75773\t48499\tMineola\tTX\tWood County\tH1\n75755\t48499\tBig sandy\tTX\tWood County\tH1\n75451\t48499\tLeesburg\tTX\tWood County\tH1\n75494\t48499\tWinnsboro\tTX\tWood County\tH1\n75471\t48499\tPickton\tTX\tWood County\tH1\n75783\t48499\tQuitman\tTX\tWood County\tH1\n75444\t48499\tGolden\tTX\tWood County\tH1\n79376\t48501\tTokio\tTX\tYoakum County\tH1\n79360\t48501\tSeminole\tTX\tYoakum County\tH1\n79323\t48501\tDenver city\tTX\tYoakum County\tH1\n79355\t48501\tPlains\tTX\tYoakum County\tH1\n76424\t48503\tBreckenridge\tTX\tYoung County\tH1\n76372\t48503\tNewcastle\tTX\tYoung County\tH1\n76481\t48503\tSouth bend\tTX\tYoung County\tH1\n76460\t48503\tLoving\tTX\tYoung County\tH1\n76374\t48503\tOlney\tTX\tYoung County\tH1\n76491\t48503\tWoodson\tTX\tYoung County\tH1\n76427\t48503\tBryson\tTX\tYoung County\tH1\n76450\t48503\tGraham\tTX\tYoung County\tH1\n76389\t48503\tWindthorst\tTX\tYoung County\tH1\n78584\t48505\tRoma\tTX\tZapata County\tH1\n78076\t48505\tZapata\tTX\tZapata County\tH1\n78360\t48505\tGuerra\tTX\tZapata County\tH1\n78067\t48505\tSan ygnacio\tTX\tZapata County\tH1\n78564\t48505\tLopeno\tTX\tZapata County\tH1\n78361\t48505\tHebbronville\tTX\tZapata County\tH1\n78061\t48507\tPearsall\tTX\tZavala County\tH1\n78872\t48507\tLa pryor\tTX\tZavala County\tH1\n78834\t48507\tCarrizo springs\tTX\tZavala County\tH1\n78839\t48507\tCrystal city\tTX\tZavala County\tH1\n78829\t48507\tBatesville\tTX\tZavala County\tH1\n84752\t49001\tMinersville\tUT\tBeaver County\tH1\n84743\t49001\tKingston\tUT\tBeaver County\tH1\n84713\t49001\tBeaver\tUT\tBeaver County\tH1\n84751\t49001\tMilford\tUT\tBeaver County\tH1\n84731\t49001\tGreenville\tUT\tBeaver County\tH1\n84307\t49003\tCorinne\tUT\tBox Elder County\tH1\n84313\t49003\tGrouse creek\tUT\tBox Elder County\tH1\n84306\t49003\tCollinston\tUT\tBox Elder County\tH1\n84324\t49003\tMantua\tUT\tBox Elder County\tH1\n84302\t49003\tBrigham city\tUT\tBox Elder County\tH1\n84336\t49003\tSnowville\tUT\tBox Elder County\tH1\n84311\t49003\tFielding\tUT\tBox Elder County\tH1\n84329\t49003\tPark valley\tUT\tBox Elder County\tH1\n84316\t49003\tHowell\tUT\tBox Elder County\tH1\n84301\t49003\tBear river city\tUT\tBox Elder County\tH1\n84340\t49003\tWillard\tUT\tBox Elder County\tH1\n84314\t49003\tHoneyville\tUT\tBox Elder County\tH1\n84331\t49003\tPortage\tUT\tBox Elder County\tH1\n84312\t49003\tGarland\tUT\tBox Elder County\tH1\n84337\t49003\tTremonton\tUT\tBox Elder County\tH1\n84309\t49003\tDeweyville\tUT\tBox Elder County\tH1\n84330\t49003\tPlymouth\tUT\tBox Elder County\tH1\n84334\t49003\tRiverside\tUT\tBox Elder County\tH1\n84321\t49005\tLogan\tUT\tCache County\tH1\n84323\t49005\tLogan\tUT\tCache County\tH1\n84335\t49005\tSmithfield\tUT\tCache County\tH1\n84326\t49005\tMillville\tUT\tCache County\tH1\n84333\t49005\tRichmond\tUT\tCache County\tH1\n84304\t49005\tCache junction\tUT\tCache County\tH1\n84327\t49005\tNewton\tUT\tCache County\tH1\n84308\t49005\tCornish\tUT\tCache County\tH1\n84339\t49005\tWellsville\t
